vi "AngleWrapper.vi"(0 "Heading In (rad)":dbl) -> (1 "Heading Out (rad)":dbl, 2 "Heading Out (deg)":dbl)   [LabVIEW 2011]
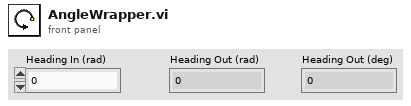
[diagram p1: front panel]
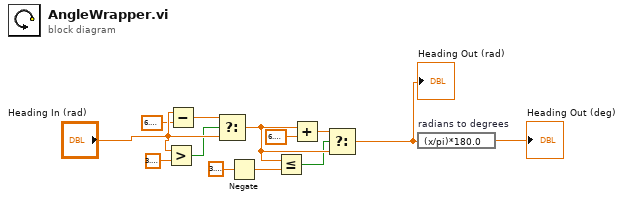
[diagram p0: block diagram]
diagram:
  n1 = Greater?(x="Heading In (rad)", y=3.141592653589793) -> (0:w6:bool)
  n2 = Subtract(x="Heading In (rad)", y=6.283185307179586) -> (x-y=w10:dbl)
  n3 = Select(t=w10, s=w6, f="Heading In (rad)") -> (s? t:f=w9:dbl)
  n4 = Negate(x=3.141592653589793) -> (-x=w1:dbl)
  n5 = Less Or Equal?(x=w9, y=w1) -> (x <= y?=w7:bool)
  n6 = Add(x=w9, y=6.283185307179586) -> (x+y=w8:dbl)
  n7 = Select(t=w8, s=w7, f=w9) -> (s? t:f=w12:dbl)
  "Heading Out (rad)" <- w12
  n8 = expression code="(x/pi)*180.0" "radians to degrees"(w12) -> (→"Heading Out (deg)":dbl)
